vi "Flush.vi"(8 "error in (no error)":errorcluster, 11 "name":string) -> (0 "error out":errorcluster)   [LabVIEW 2017, in "DVRBuffer.lvlib"]
uses:
  <vilib>/addons/InsightCM/Devices/Shared/Common/DVRBuffer/DVRBuffer.lvlib
  <vilib>/addons/InsightCM/Devices/Shared/Common/DVRBuffer/controls/DVRElement.ctl
  <vilib>/addons/InsightCM/Devices/Shared/Common/DVRBuffer/controls/InternalDataType_waveformmap.ctl
  <vilib>/addons/PointValueMap/controls/PointMap.ctl
  <vilib>/addons/PointValueMap/PointValueMap.lvlib
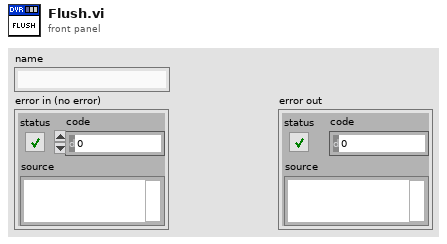
[diagram p1: front panel]
types:
  T1 = typedef "DVRBuffer.lvlib/DVRBuffer.ctl" = cluster{"buffer":T2[], "write ptr index":i32, "last block":u32, "buffer size":u32}
  T2 = typedef "DVRBuffer.lvlib/DVRElement.ctl" = cluster{"location":u32, "DVR":u32, "points":i32, "dt":dbl, "PulsePositions":dbl[], "Pulses Per Rev":dbl}
  T3 = typedef "DVRBuffer.lvlib/InternalDataType_waveformmap.ctl" = cluster{"waveforms":waveform(sgl)[], "map":T4}
  T4 = typedef "PointValueMap.lvlib/PointMap.ctl" = refnum<data-value>
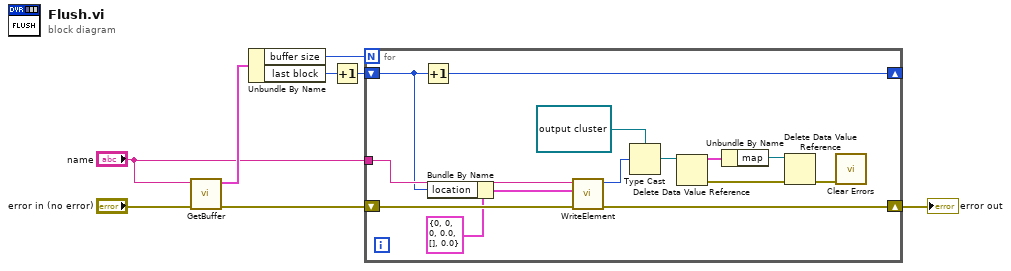
[diagram p0: block diagram]
diagram:
  n1 = call <vilib>:"GetBuffer.vi"("error in (no error)"="error in (no error)", "name"="name") -> ("error out"=w5:errorcluster, "DVRBuffer"=w7:T1)  [unwired: 8 in]
  n2 = Unbundle By Name(w7) -> ("buffer size"=w6:u32, "last block"=w2:u32)
  n3 = Increment(x=w2) -> (x+1=w1:u32)
  n4 = for {
    N: w6 -> [_]
    tunnel: "name" -> [w21]
    shift-right: [w13] -> w3
    shift-left: w5 -> [w22]
    shift-right: [w9] -> _
    shift-left: w1 -> [w10]
    n5 = Increment(x=w10) -> (x+1=w9:u32)
    n6 = Bundle By Name(cluster=T2 {"location"=0, "DVR"=0, "points"=0, "dt"=0.0, "PulsePositions"=[], "Pulses Per Rev"=0.0} ("dvr element"), "location"=w10) -> (w11:T2)
    n7 = call <vilib>:"WriteElement.vi"("error in (no error)"=w22, "dvr element"=w11, "name"=w21) -> ("error out"=w13:errorcluster, "replaced dvr"=w14:u32)  [unwired: 6 in, 1 out]
    n8 = Type Cast(type=refnum<data-value> refnum ("data value reference"), x=w14) -> (*(type *) &x=w20:refnum<data-value>)
    n9 = Delete Data Value Reference(data value reference=w20) -> (data value=w19:T3, error out=w17:errorcluster)  [unwired: 1 in]
    n10 = Unbundle By Name(w19) -> ("map"=w18:T4)
    n11 = Delete Data Value Reference(data value reference=w18, error in=w17) -> (error out=w16:errorcluster)  [unwired: 1 out]
    n12 = call <vilib>:"Clear Errors.vi"("error in (no error)"=w16) -> ()  [unwired: 5 in, 2 out]
  }
  "error out" <- w3
